vi "prep.vi"(8 "error in (no error)":errorcluster, 9 "Coordinate System":enum16{"Cartesian", "Cylindrical", "Spherical"}(ring), 10 "Plot processed data In":T1 caption="Data In", 11 "Line in":refnum<class "Line.lvclass">) -> (0 "error out":errorcluster, 2 "Plot processed Data Out":T1 caption="Data Out", 3 "Line out":refnum<class "Line.lvclass">)   [LabVIEW 2020, in "Line.lvclass"]
uses:
  <vilib>/Native 3D Graph/classes/Line/Line.lvclass
  <vilib>/Native 3D Graph/xcontrol/Processed Data.ctl
  <vilib>/Native 3D Graph/typedefs/plot_rep_array.ctl
  <vilib>/Native 3D Graph/typedefs/plot_rep.ctl
  <vilib>/Native 3D Graph/typedefs/range_cluster.ctl
  <vilib>/Native 3D Graph/typedefs/min_max.ctl
  <vilib>/Native 3D Graph/typedefs/plot_rep_mesh_data.ctl
  <vilib>/Native 3D Graph/classes/Line/Line.lvclass/Line.ctl
  <vilib>/Analysis/coordinate.llb/3D Coordinate Conversion (Scalar).vi
  <vilib>/Native 3D Graph/classes/Base Datatype.lvclass
  <vilib>/Native 3D Graph/xcontrol/3DPC_SurfacePlot.xctl
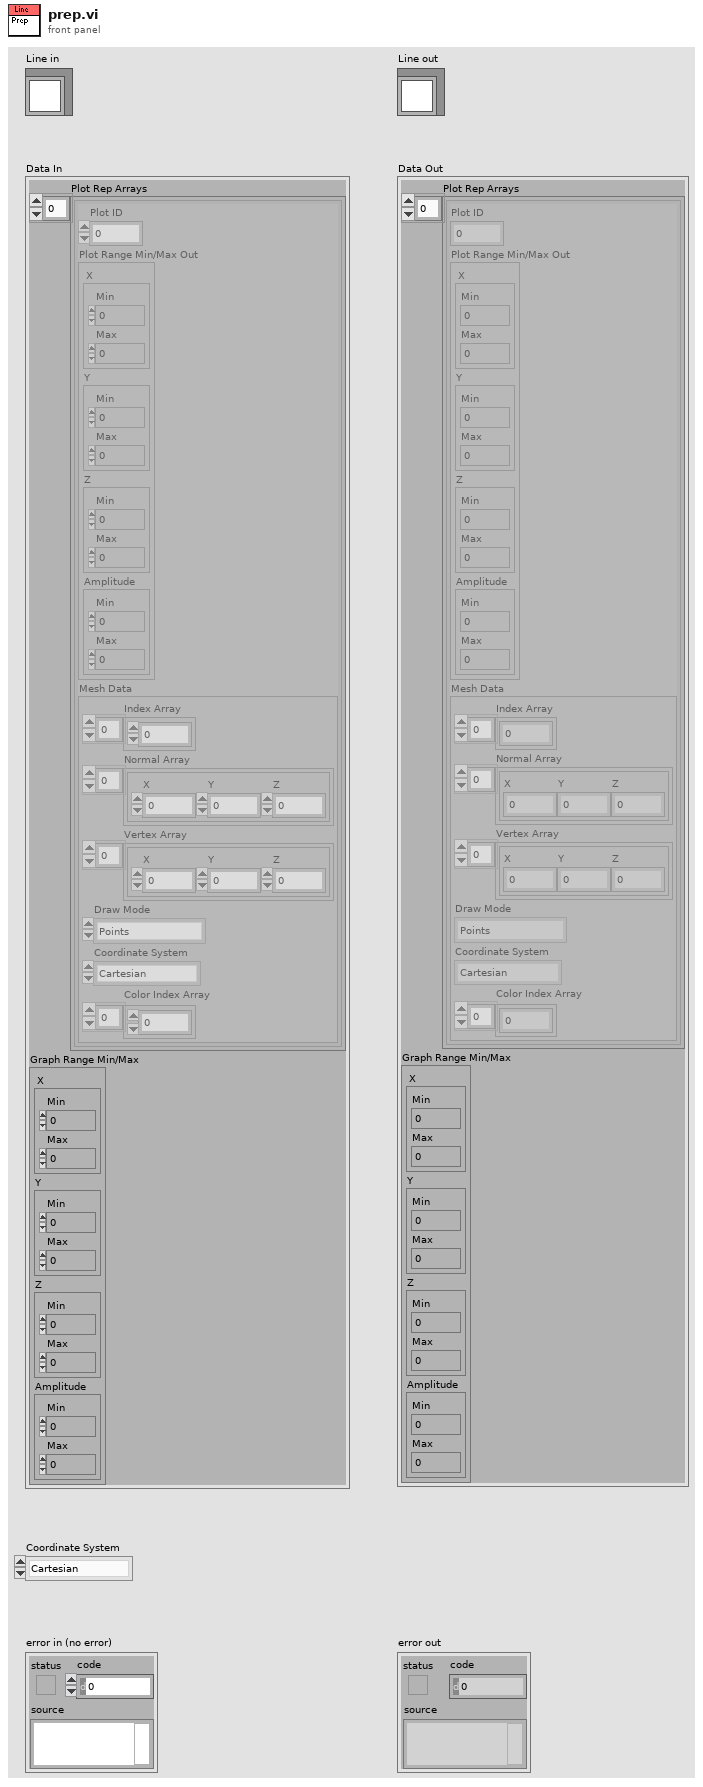
[diagram p1: front panel]
types:
  T1 = typedef "Processed Data.ctl" = cluster{"Plot Rep Arrays":T2, "Graph Range Min/Max":T4}
  T2 = typedef "3DPC_SurfacePlot.xctl/plot_rep_array.ctl" = T3[]
  T3 = typedef "3DPC_SurfacePlot.xctl/plot_rep.ctl" = cluster{"Plot ID":i32, "Plot Range Min/Max Out":T4, "Mesh Data":T6}
  T4 = typedef "3DPC_SurfacePlot.xctl/range_cluster.ctl" = cluster{"X":T5, "Y":T5, "Z":T5, "Amplitude":T5}
  T5 = typedef "3DPC_SurfacePlot.xctl/min_max.ctl" = cluster{"Min":sgl, "Max":sgl}
  T6 = typedef "3DPC_SurfacePlot.xctl/plot_rep_mesh_data.ctl" = cluster{"Index Array":u32[], "Normal Array":cluster{"X":sgl, "Y":sgl, "Z":sgl}[], "Vertex Array":cluster{"X":sgl, "Y":sgl, "Z":sgl}[], "Draw Mode":enum16{"Points", "Lines", "Line Strip", "Line Loop", "Triangles", "Triangle Strip", "Triangle Fan", "Quads", "Quad Strip", "Polygon"}, "Coordinate System":enum16{"Cartesian", "Cylindrical", "Spherical"}, "Color Index Array":i32[]}
  T7 = enum16{"Points", "Lines", "Line Strip", "Line Loop", "Triangles", "Triangle Strip", "Triangle Fan", "Quads", "Quad Strip", "Polygon"}
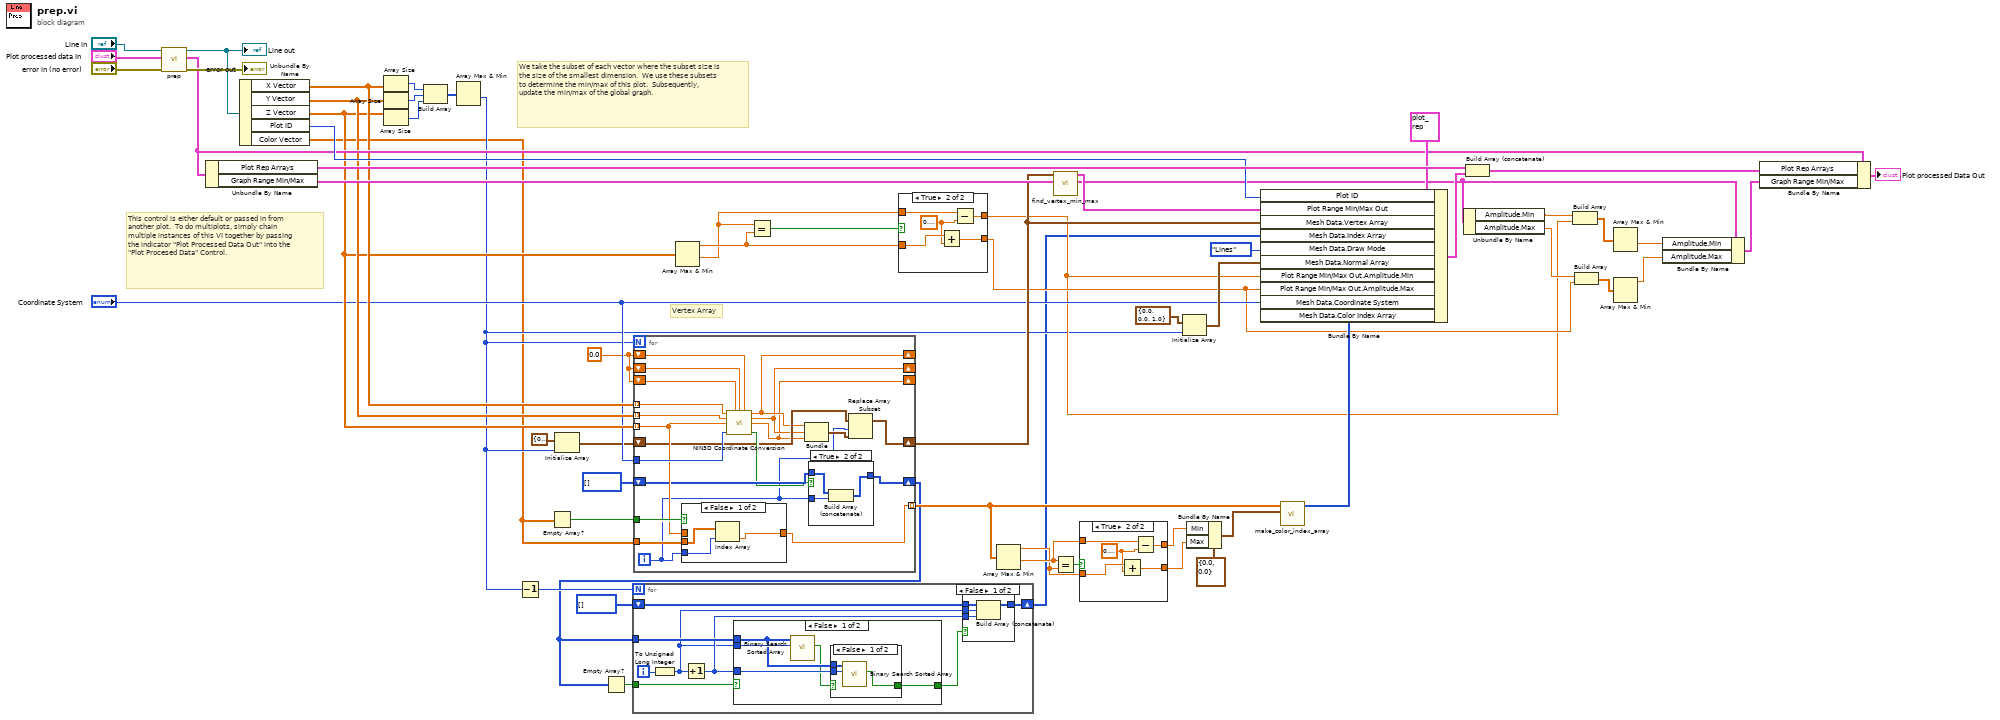
[diagram p0: block diagram]
diagram:
  w7 = sgl 0.0
  # "We take the subset of each vector where the subset size is the size of the smallest dimension.  We use these subsets to determine the min/max of this plot.  Subsequently, update the min/max of the global graph."
  # "This control is either default or passed in from another plot.  To do multiplots, simply chain multiple instances of this VI together by passing the indicator \"Plot Processed Data Out\" into the \"Plot Procesed Data\" Control."
  # "Vertex Array"
  n1 = call-parent "prep.vi"("error in (no error)"="error in (no error)", "Plot processed data In"="Plot processed data In", "Base Datatype in"="Line in") -> ("error out"=→"error out":errorcluster, "Plot processed Data Out"=w42:T1, "Base Datatype out"=w56:refnum<class "Line.lvclass">)  [unwired: 1 in, 5 out]
  "Line out" <- w56
  n2 = Unbundle By Name(w42) -> ("Plot Rep Arrays"=w55:T2, "Graph Range Min/Max"=w40:T4)
  n3 = Unbundle By Name(w56) -> ("X Vector"=w38:sgl[], "Y Vector"=w37:sgl[], "Z Vector"=w35:sgl[], "Plot ID"=w43:i32, "Color Vector"=w2:sgl[])
  n4 = Array Size(array=w38) -> (size(s)=w52:i32)
  n5 = Array Size(array=w37) -> (size(s)=w51:i32)
  n6 = Array Size(array=w35) -> (size(s)=w50:i32)
  n7 = Build Array(w52, w51, w50) -> (w49:i32[])
  n8 = Array Max & Min(array=w49) -> (min value=w10:i32)  [unwired: 3 out]
  n9 = Decrement(x=w10) -> (x-1=w44:i32)
  n10 = Empty Array?(array=w2) -> (empty?=w3:bool)
  n11 = Initialize Array(cluster{"X":sgl, "Y":sgl, "Z":sgl} {"X"=0.0, "Y"=0.0, "Z"=0.0} ("3D Point"), w10) -> (w8:cluster{"X":sgl, "Y":sgl, "Z":sgl}[])
  n12 = for {
    N: w10 -> [_]
    shift-right: [w69] -> w36
    shift-left: w8 -> [w70]
    tunnel: w38 -> [w80] mode=indexing
    tunnel: w37 -> [w79] mode=indexing
    tunnel: w35 -> [w76] mode=indexing
    tunnel: "Coordinate System" -> [w78]
    tunnel: w3 -> [w77]
    tunnel: [w74] -> w17 mode=indexing
    tunnel: w2 -> [w75]
    shift-right: [w71] -> w6
    shift-left: u32[] [] -> [w73]
    shift-right: [w63] -> _
    shift-left: w7 -> [w66]
    shift-right: [w62] -> _
    shift-left: w7 -> [w65]
    shift-right: [w61] -> _
    shift-left: w7 -> [w64]
    i -> [w67]
    n13 = case shown="False" w77 {
      tunnel: w76 -> [_ w88]
      tunnel: [w85 w88] -> w74
      tunnel: w75 -> [w86 _]
      tunnel: w67 -> [w87 _]
      frame False {
        n14 = Index Array(array=w86, index=w87) -> (element=w85:sgl)
      }
      frame True {
      }
    }
    n15 = call <vilib>:"NIN3D Coordinate Conversion.vi"("X"=w80, "Z_prev"=w64, "Y_prev"=w65, "X_prev"=w66, "Y"=w79, "Z"=w76, "Coordinate System"=w78) -> ("X out"=w63:sgl, "Y out"=w62:sgl, "Z out"=w61:sgl, "NaN?"=w72:bool)  [unwired: 5 in]
    n16 = Bundle("X out"=w63, "Y out"=w62, "Z out"=w61) -> (w68:cluster{"X out":sgl, "Y out":sgl, "Z out":sgl})  [unwired: 1 out]
    n17 = case shown="True" w72 {
      tunnel: w73 -> [w81 w84]
      tunnel: [w81 w83] -> w71
      tunnel: w67 -> [_ w82]
      frame False {
      }
      frame True {
        n18 = Build Array (concatenate)(w84, w82) -> (w83:u32[])
      }
    }
    n19 = Replace Array Subset(array=w70, new element=w68, index=w67) -> (w69:cluster{"X":sgl, "Y":sgl, "Z":sgl}[])
  }
  n20 = Empty Array?(array=w6) -> (empty?=w5:bool)
  n21 = for {
    N: w44 -> [_]
    shift-right: [w95] -> w4
    shift-left: u32[] [] ("Indices") -> [w96]
    tunnel: w6 -> [w93]
    tunnel: w5 -> [w91]
    i -> [w90]
    n22 = To Unsigned Long Integer(number=w90) -> (unsigned 32bit integer=w89:u32)
    n23 = Increment(x=w89) -> (x+1=w92:u32)
    n24 = case shown="False" w91 {
      tunnel: [w102 _] -> w94
      tunnel: w93 -> [w104 _]
      tunnel: w89 -> [w106 _]
      tunnel: w92 -> [w105 _]
      frame False {
        n25 = call <vilib>:"Binary Search Sorted Array.vi"("Element"=w106, "Sorted Array"=w104) -> ("Found?"=w103:bool)  [unwired: 9 in]
        n26 = case shown="False" w103 {
          selector: w103 -> [_ w110]
          tunnel: w105 -> [w109 _]
          tunnel: w104 -> [w108 _]
          tunnel: [w107 w110] -> w102
          frame False {
            n27 = call <vilib>:"Binary Search Sorted Array.vi"("Element"=w109, "Sorted Array"=w108) -> ("Found?"=w107:bool)  [unwired: 9 in]
          }
          frame True {
          }
        }
      }
      frame True {
      }
    }
    n28 = case shown="False" w94 {
      tunnel: w96 -> [w100 w101]
      tunnel: [w99 w101] -> w95
      tunnel: w92 -> [w98 _]
      tunnel: w89 -> [w97 _]
      frame False {
        n29 = Build Array (concatenate)(w100, w97, w98) -> (w99:u32[])
      }
      frame True {
      }
    }
  }
  n30 = Array Max & Min(array=w35) -> (max value=w19:sgl, min value=w18:sgl)  [unwired: 2 out]
  n31 = Equal?(x=w18, y=w19) -> (x = y?=w22:bool)
  n32 = case shown="True" w22 {
    tunnel: w19 -> [w112 w117]
    tunnel: [w112 w116] -> w21
    tunnel: w18 -> [w111 w115]
    tunnel: [w111 w114] -> w20
    frame False {
    }
    frame True {
      w113 = sgl 0.1 ("y")
      n33 = Add(x=w117, y=w113) -> (x+y=w116:sgl)
      n34 = Subtract(x=w115, y=w113) -> (x-y=w114:sgl)
    }
  }
  n35 = Array Max & Min(array=w17) -> (max value=w13:sgl, min value=w14:sgl)  [unwired: 2 out]
  n36 = call <vilib>:"find_vertex_min_max.vi"("Total Range Min/Max"=w40, "Vertex Array"=w36) -> ("Total Range Out"=w27:T4, "This Range Min/Max Out"=w39:T4)  [unwired: 8 out]
  n37 = Equal?(x=w14, y=w13) -> (x = y?=w12:bool)
  n38 = case shown="True" w12 {
    tunnel: w13 -> [w119 w124]
    tunnel: [w119 w123] -> w15
    tunnel: w14 -> [w118 w122]
    tunnel: [w118 w121] -> w16
    frame False {
    }
    frame True {
      w120 = sgl 0.1 ("y")
      n39 = Add(x=w124, y=w120) -> (x+y=w123:sgl)
      n40 = Subtract(x=w122, y=w120) -> (x-y=w121:sgl)
    }
  }
  n41 = Initialize Array(cluster{"X":sgl, "Y":sgl, "Z":sgl} {"X"=0.0, "Y"=0.0, "Z"=1.0} ("3D Point"), w10) -> (w45:cluster{"X":sgl, "Y":sgl, "Z":sgl}[])
  n42 = Bundle By Name(cluster=T5 {"Min"=0.0, "Max"=0.0} ("Amplitude"), "Min"=w16, "Max"=w15) -> (w24:T5)
  n43 = call <vilib>:"make_color_index_array.vi"("Amplitude Min/Max"=w24, "Z array"=w17) -> ("Color Index Array"=w23:i32[])  [unwired: 9 out]
  n44 = Bundle By Name(cluster=T3 {"Plot ID"=0, "Plot Range Min/Max Out"={"X"={"Min"=0.0, "Max"=0.0}, "Y"={"Min"=0.0, "Max"=0.0}, "Z"={"Min"=0.0, "Max"=0.0}, "Amplitude"={"Min"=0.0, "Max"=0.0}}, "Mesh Data"={"Index Array"=[], "Normal Array"=[], "Vertex Array"=[], "Draw Mode"=enum."Points", "Coordinate System"=enum."Cartesian", "Color Index Array"=[]}} ("Plot Representation"), "Plot ID"=w43, "Plot Range Min/Max Out"=w39, "Mesh Data.Vertex Array"=w36, "Mesh Data.Index Array"=w4, "Mesh Data.Draw Mode"=T7."Lines", "Mesh Data.Normal Array"=w45, "Plot Range Min/Max Out.Amplitude.Min"=w20, "Plot Range Min/Max Out.Amplitude.Max"=w21, "Mesh Data.Coordinate System"="Coordinate System", "Mesh Data.Color Index Array"=w23) -> (w54:T3)
  n45 = Unbundle By Name(w27) -> ("Amplitude.Min"=w33:sgl, "Amplitude.Max"=w30:sgl)
  n46 = Build Array (concatenate)(w55, w54) -> (w53:T2)
  n47 = Build Array(w33, w20) -> (w32:sgl[])
  n48 = Build Array(w30, w21) -> (w29:sgl[])
  n49 = Array Max & Min(array=w32) -> (min value=w31:sgl)  [unwired: 3 out]
  n50 = Array Max & Min(array=w29) -> (max value=w28:sgl)  [unwired: 3 out]
  n51 = Bundle By Name(cluster=w27, "Amplitude.Min"=w31, "Amplitude.Max"=w28) -> (w26:T4)
  n52 = Bundle By Name(cluster=w42, "Plot Rep Arrays"=w53, "Graph Range Min/Max"=w26) -> (→"Plot processed Data Out":T1)
